vi "readBinaryFile.vi"() -> ()   [LabVIEW 2012]
panel:
  out "concatenated string":string
  in  "base path":path
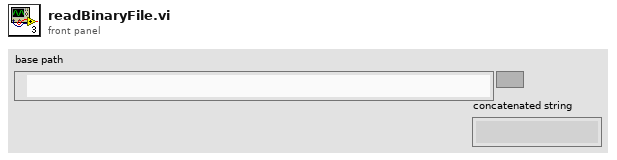
[diagram p1: front panel]
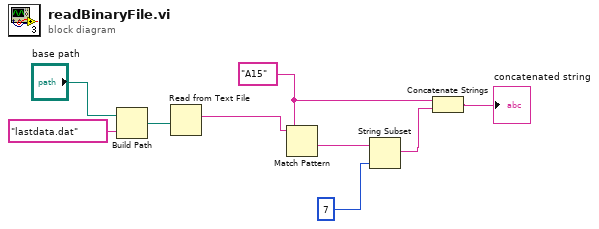
[diagram p0: block diagram]
diagram:
  w3 = "A15" ("regular expression")
  n1 = Build Path(base path="base path", name or relative path="lastdata.dat") -> (appended path=w9:path)
  n2 = Read from Text File(file (use dialog)=w9) -> (text=w6:string)  [unwired: 3 in, 3 out]
  n3 = Match Pattern(string=w6, regular expression=w3) -> (after substring=w5:string)  [unwired: 1 in, 3 out]
  n4 = String Subset(string=w5, length (rest)=7 ("length (rest)")) -> (substring=w2:string)  [unwired: 1 in]
  n5 = Concatenate Strings(w3, w2) -> (→"concatenated string":string)
